vi "Read List.vi"(0 "FILE":string, 1 "error in":errorcluster) -> (2 "output cluster":cluster{string[], string[], bool[]}, 3 "String":string, 4 "error out":errorcluster)   [LabVIEW 2018]
panel:
  out "appended path 2":path
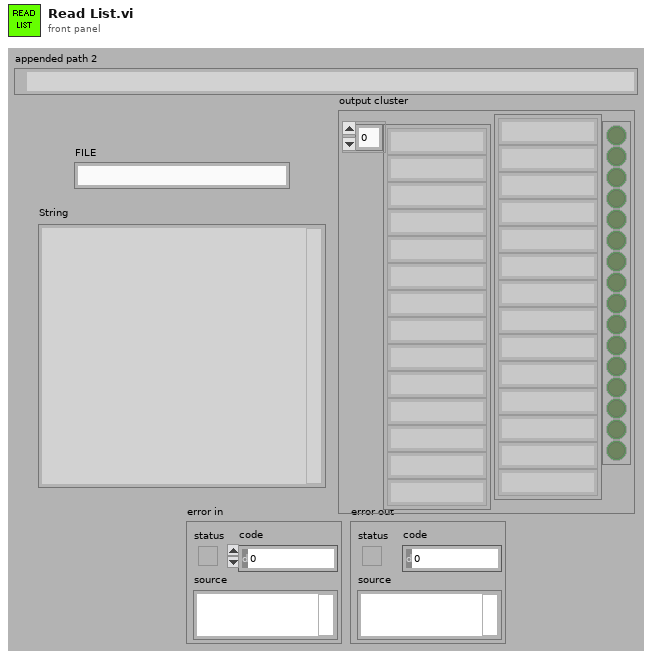
[diagram p1: front panel]
types:
  T1 = enum16{"open", "replace", "create", "open or create", "replace or create", "replace or create with confirmation"}
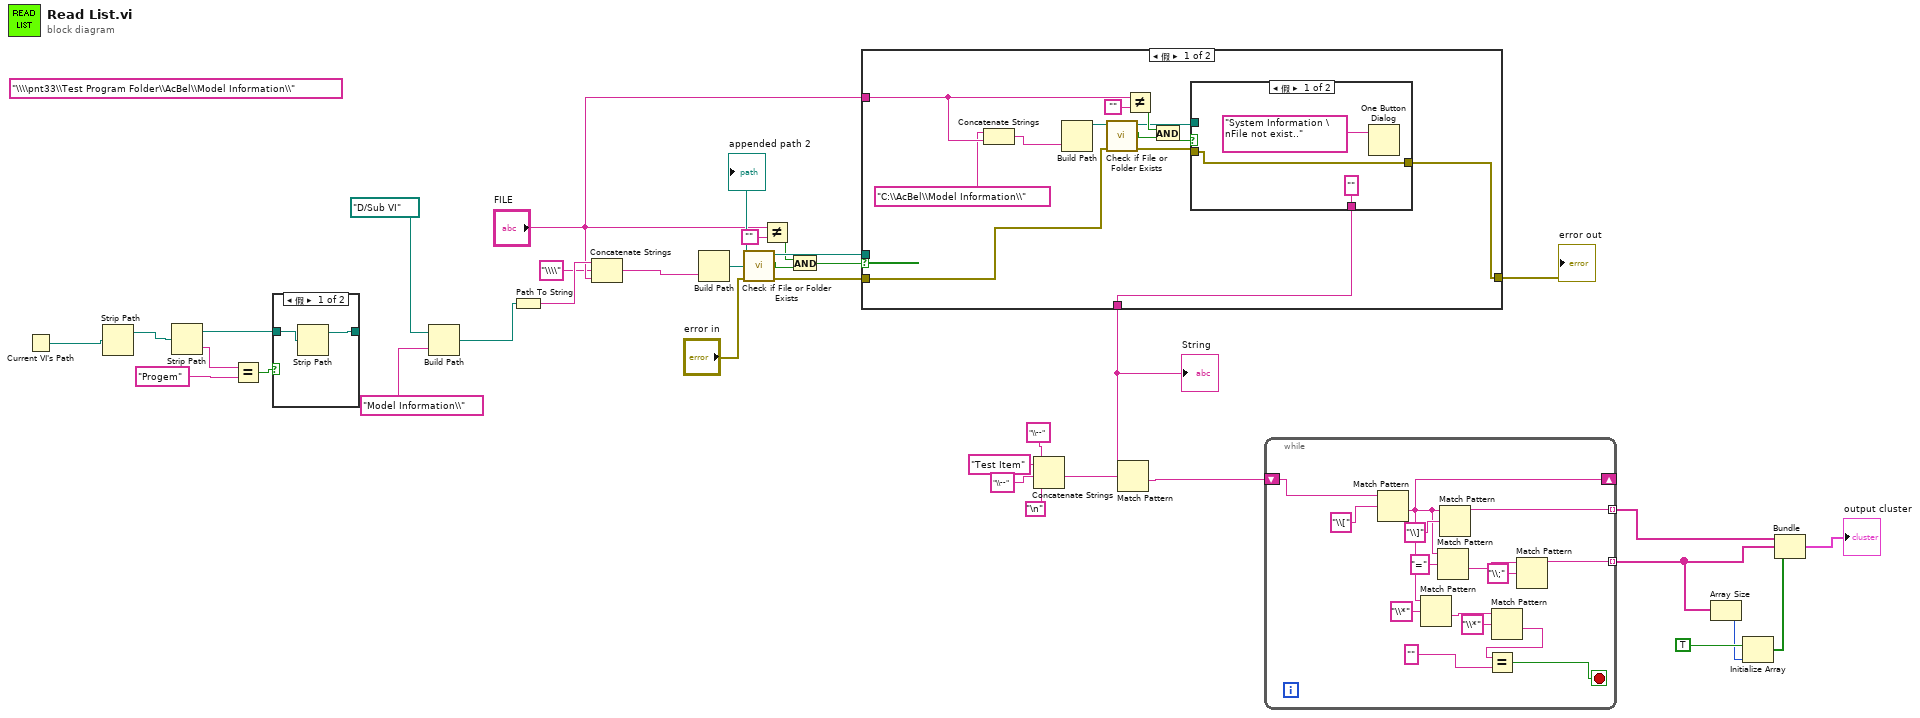
[diagram p0: block diagram]
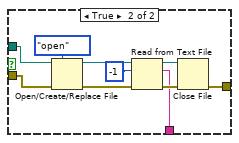
[diagram p3: hidden frame]
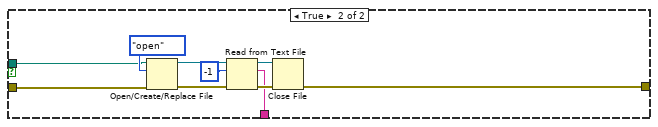
[diagram p4: hidden frame]
diagram:
  (unwired) "\\\\pnt33\\Test Program Folder\\AcBel\\Model Information\\" ("string")
  n1 = Current VI's Path() -> (path=w12:path)
  n2 = Strip Path(path=w12) -> (stripped path=w11:path)  [unwired: 1 out]
  n3 = Strip Path(path=w11) -> (stripped path=w5:path, name=w7:string)
  n4 = Equal?(x=w7, y="Progem") -> (x = y?=w4:bool)
  n5 = case shown="假" w4 {
    tunnel: w5 -> [w37 w38]
    tunnel: [w36 w38] -> _
    frame False {
      n6 = Strip Path(path=w37) -> (stripped path=w36:path)  [unwired: 1 out]
    }
    frame True {
    }
  }
  n7 = Build Path(base path=path "D:/Sub VI", name or relative path="Model Information\\") -> (appended path=w9:path)
  n8 = Path To String(path=w9) -> (string=w8:string)
  n9 = Concatenate Strings(w8, "\\\\" ("string"), "FILE") -> (w35:string)
  n10 = Build Path(name or relative path=w35) -> (appended path=w34:path)  [unwired: 1 in]
  "appended path 2" <- w34
  n11 = call <vilib>:"Check if File or Folder Exists.vi"("error in (no error)"="error in", "path"=w34) -> ("error out"=w32:errorcluster, "file or folder exists?"=w30:bool, "dup path"=w33:path)  [unwired: 7 in]
  n12 = Not Equal?(x="FILE", y="") -> (x != y?=w29:bool)
  n13 = And(x=w29, y=w30) -> (x .and. y?=w22:bool)
  n14 = case shown="假" w22 {
    tunnel: [w42 w71] -> w13
    tunnel: w33 -> [_ w65]
    tunnel: w32 -> [w40 w67]
    tunnel: [w39 w66] -> w24
    tunnel: "FILE" -> [w46 _]
    frame False {
      n15 = Concatenate Strings("C:\\AcBel\\Model Information\\" ("string"), w46) -> (w47:string)
      n16 = Build Path(name or relative path=w47) -> (appended path=w48:path)  [unwired: 1 in]
      n17 = call <vilib>:"Check if File or Folder Exists.vi"("error in (no error)"=w40, "path"=w48) -> ("error out"=w43:errorcluster, "file or folder exists?"=w50:bool, "dup path"=w44:path)  [unwired: 7 in]
      n18 = Not Equal?(x=w46, y="") -> (x != y?=w51:bool)
      n19 = And(x=w51, y=w50) -> (x .and. y?=w45:bool)
      n20 = case shown="假" w45 {
        tunnel: w44 -> [_ w58]
        tunnel: w43 -> [w52 w57]
        tunnel: ["" w56] -> w42
        tunnel: [w52 w55] -> w39
        frame False {
          n21 = One Button Dialog(message="System Information \nFile not exist..") -> ()  [unwired: 1 in, 1 out]
        }
        frame True {
          n22 = Open/Create/Replace File(file path (use dialog)=w58, error in=w57, operation (0:open)=T1."open") -> (refnum out=w62:refnum<file>, error out=w63:errorcluster)  [unwired: 3 in, 1 out]
          n23 = Read from Text File(file (use dialog)=w62, count=-1, error in=w63) -> (refnum out=w61:refnum<file>, text=w56:string, error out=w60:errorcluster)  [unwired: 1 in, 1 out]
          n24 = Close File(refnum=w61, error in=w60) -> (error out=w55:errorcluster)  [unwired: 1 out]
        }
      }
    }
    frame True {
      n25 = Open/Create/Replace File(file path (use dialog)=w65, error in=w67, operation (0:open)=T1."open") -> (refnum out=w70:refnum<file>, error out=w69:errorcluster)  [unwired: 3 in, 1 out]
      n26 = Read from Text File(file (use dialog)=w70, count=-1, error in=w69) -> (refnum out=w72:refnum<file>, text=w71:string, error out=w73:errorcluster)  [unwired: 1 in, 1 out]
      n27 = Close File(refnum=w72, error in=w73) -> (error out=w66:errorcluster)  [unwired: 1 out]
    }
  }
  "error out" <- w24
  "String" <- w13
  n28 = Concatenate Strings("\\--" ("regular expression"), "Test Item" ("string"), "\\--" ("string"), "\n") -> (w28:string)
  n29 = Match Pattern(string=w13, regular expression=w28) -> (after substring=w20:string)  [unwired: 1 in, 3 out]
  n30 = while {
    tunnel: [w87] -> w15 mode=indexing
    shift-right: [w78] -> _
    shift-left: w20 -> [w79]
    tunnel: [w83] -> w17 mode=indexing
    stop <- w81 stop-if-true
    n31 = Match Pattern(string=w79, regular expression="\\[") -> (after substring=w78:string)  [unwired: 1 in, 3 out]
    n32 = Match Pattern(string=w78, regular expression="\\*") -> (after substring=w76:string)  [unwired: 1 in, 3 out]
    n33 = Match Pattern(string=w78, regular expression="=") -> (after substring=w85:string)  [unwired: 1 in, 3 out]
    n34 = Match Pattern(string=w78, regular expression="\\]" ("string")) -> (before substring=w87:string)  [unwired: 1 in, 3 out]
    n35 = Match Pattern(string=w76, regular expression="\\*") -> (after substring=w75:string)  [unwired: 1 in, 3 out]
    n36 = Equal?(x=w75, y="") -> (x = y?=w81:bool)
    n37 = Match Pattern(string=w85, regular expression="\\;") -> (before substring=w83:string)  [unwired: 1 in, 3 out]
  }
  n38 = Array Size(array=w17) -> (size(s)=w18:i32)
  n39 = Initialize Array(TRUE, w18) -> (w16:bool[])
  n40 = Bundle(w15, w17, w16) -> (→"output cluster":cluster{string[], string[], bool[]})  [unwired: 1 in]
